vi "Drive_Teleop.vi"(11 "Joystick_In":T1) -> ()   [LabVIEW 2019]
uses:
  Utility_VIs/Joystick_Controls.ctl
  Subsystems/Drive/Drive_Cluster.ctl
  Subsystems/Drive/Drive_States.ctl
  Globals/Drive_Globals.vi
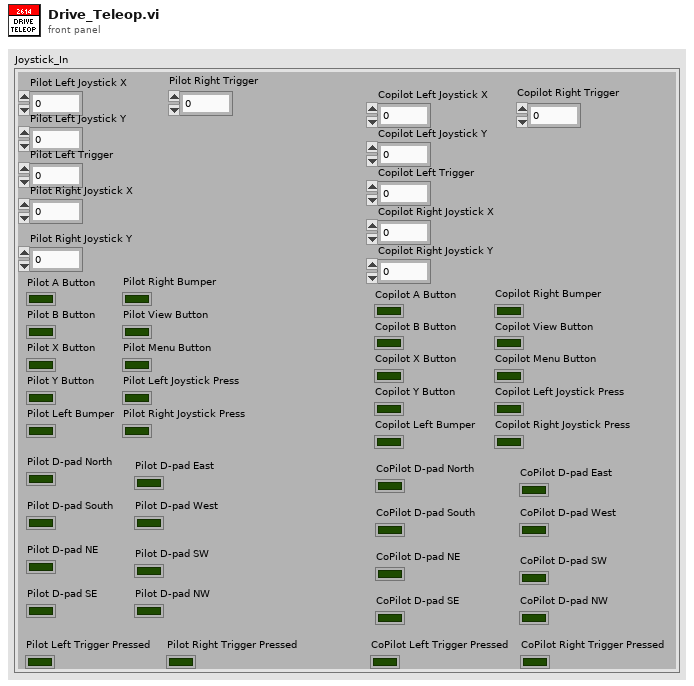
[diagram p1: front panel]
types:
  T1 = typedef "Joystick_Controls.ctl" = cluster{"Pilot Left Joystick X":dbl, "Pilot Left Joystick Y":dbl, "Pilot A Button":bool, "Pilot B Button":bool, "Pilot X Button":bool, "Pilot Y Button":bool, "Pilot Left Bumper":bool, "Pilot Right Bumper":bool, "Pilot View Button":bool, "Pilot Menu Button":bool, "Pilot Left Joystick Press":bool, "Pilot Right Joystick Press":bool, "Pilot Left Trigger":dbl, "Pilot Right Joystick X":dbl, "Pilot Right Joystick Y":dbl, "Pilot Right Trigger":dbl, "Copilot Left Joystick X":dbl, "Copilot Left Joystick Y":dbl, "Copilot A Button":bool, "Copilot B Button":bool, "Copilot X Button":bool, "Copilot Y Button":bool, "Copilot Left Bumper":bool, "Copilot Right Bumper":bool, "Copilot View Button":bool, "Copilot Menu Button":bool, "Copilot Left Joystick Press":bool, "Copilot Right Joystick Press":bool, "Copilot Left Trigger":dbl, "Copilot Right Joystick X":dbl, "Copilot Right Joystick Y":dbl, "Copilot Right Trigger":dbl, "Pilot D-pad North":bool, "Pilot D-pad South":bool, "Pilot D-pad East":bool, "Pilot D-pad West":bool, "Pilot D-pad NE ":bool, "Pilot D-pad SE":bool, "Pilot D-pad SW":bool, "Pilot D-pad NW":bool, "CoPilot D-pad North":bool, "CoPilot D-pad South":bool, "CoPilot D-pad East":bool, "CoPilot D-pad West":bool, "CoPilot D-pad NE":bool, "CoPilot D-pad SE":bool, "CoPilot D-pad SW":bool, "CoPilot D-pad NW":bool, "Pilot Left Trigger Pressed":bool, "Pilot Right Trigger Pressed":bool, "CoPilot Left Trigger Pressed":bool, "CoPilot Right Trigger Pressed":bool}
  T2 = typedef "Drive_Cluster.ctl" = cluster{"Control_State":T3, "Angular_Throttle":dbl, "Linear_Throttle":dbl, "Torque_Changing":bool}
  T3 = typedef "Drive_States.ctl" = enum16{"Percent_Voltage_Control", "Speed_Control"}
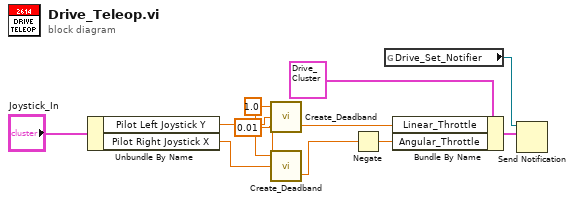
[diagram p0: block diagram]
diagram:
  w3 = 1.0 ("Output Upper Limit")
  w2 = 0.01 ("Output Lower Limit")
  n1 = Unbundle By Name("Joystick_In") -> ("Pilot Left Joystick Y"=w6:dbl, "Pilot Right Joystick X"=w4:dbl)
  n2 = call "Create_Deadband.vi"("Output Lower Limit"=w2, "Input"=w6, "Output Upper Limit"=w3) -> ("Output"=w5:dbl)  [unwired: 1 out]
  n3 = call "Create_Deadband.vi"("Output Lower Limit"=w2, "Input"=w4, "Output Upper Limit"=w3) -> ("Output"=w1:dbl)  [unwired: 1 out]
  n4 = Negate(x=w1) -> (-x=w7:dbl)
  n5 = global read "Drive_Globals.vi" "Drive_Set_Notifier"() -> (w11:refnum<notifier>)
  n6 = Bundle By Name(cluster=T2 {"Control_State"=enum."Percent_Voltage_Control", "Angular_Throttle"=0.0, "Linear_Throttle"=0.0, "Torque_Changing"=FALSE} ("notification"), "Linear_Throttle"=w5, "Angular_Throttle"=w7) -> (w9:T2)
  n7 = Send Notification(notification=w9, notifier=w11) -> ()  [unwired: 1 in, 2 out]
